vi "addSuccess.vi"(7 "execution time (sec)":dbl, 8 "error in (no error)":errorcluster, 10 "test":refnum<class>, 11 "TestResult in":refnum<class "TestResult.lvclass">) -> (0 "error out":errorcluster, 3 "TestResult in":refnum<class "TestResult.lvclass">)   [LabVIEW 2019, in "TestResult.lvclass"]
uses:
  TestResult.lvclass
  resultStatusChanged--Cluster.ctl
  resultStatus--enum.ctl
  TestResult.lvclass/TestResult.ctl
panel:
  # "JKI VI Tester for LabVIEW\nhttp://jkisoft.com/vi-tester\nCopyright (C) 2007-2009, JKI <info@jkisoft.com>\nALL RIGHTS RESERVED"
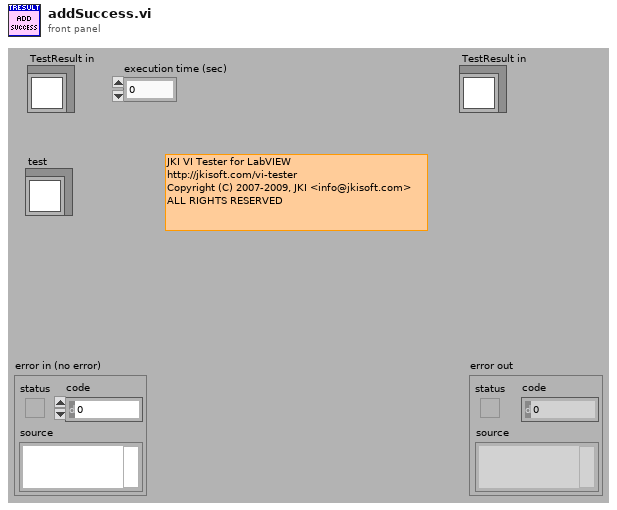
[diagram p1: front panel]
types:
  T1 = typedef "TestResult.lvclass/resultStatusChanged--Cluster.ctl" = cluster{"test":refnum<class>, "resultStatus":T2, "TestResult":refnum<class>, "test error":errorcluster, "execution time (sec)":dbl}
  T2 = typedef "TestResult.lvclass/resultStatus--enum.ctl" = enum16{"testPass", "testFailure", "testError", "testSkipped"}
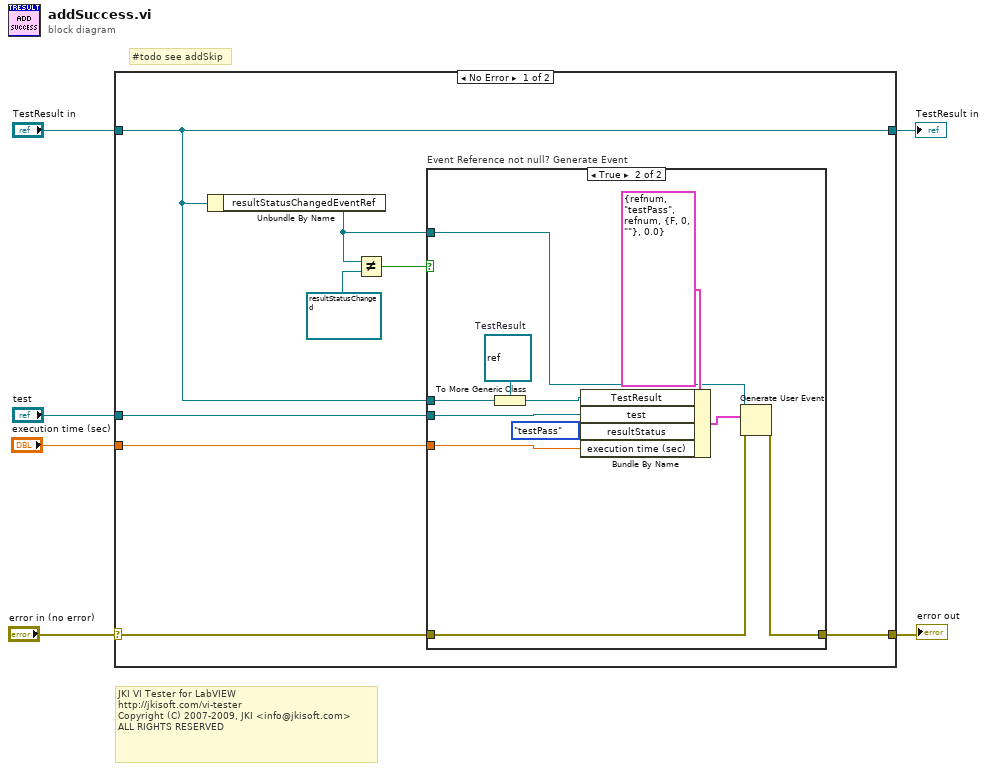
[diagram p0: block diagram]
diagram:
  # "#todo see addSkip"
  # "JKI VI Tester for LabVIEW\nhttp://jkisoft.com/vi-tester\nCopyright (C) 2007-2009, JKI <info@jkisoft.com>\nALL RIGHTS RESERVED"
  n1 = case shown="No Error" "error in (no error)" {
    selector: "error in (no error)" -> [w10 w28]
    tunnel: [w9 w28] -> w5
    tunnel: [w13 w27] -> w3
    tunnel: "TestResult in" -> [w13 w27]
    tunnel: "test" -> [w14 _]
    tunnel: "execution time (sec)" -> [w7 _]
    frame No Error {
      n2 = Unbundle By Name(w13) -> ("resultStatusChangedEventRef"=w12:refnum<user-event>)
      n3 = Not Equal?(x=w12, y=refnum<user-event> refnum ("resultStatusChangedEventRef")) -> (x != y?=w8:bool)
      n4 = case "Event Reference not null? Generate Event" shown="True" w8 {
        tunnel: w14 -> [_ w24]
        tunnel: w13 -> [_ w23]
        tunnel: w12 -> [_ w21]
        tunnel: w10 -> [w15 w20]
        tunnel: [w15 w19] -> w9
        tunnel: w7 -> [_ w16]
        frame False {
        }
        frame True {
          w17 = refnum<class> refnum  # TestResult
          n5 = To More Generic Class(target class=w17, reference=w23) -> (generic class reference=w18:refnum<class>)
          n6 = Bundle By Name(cluster=T1 {"test"=refnum, "resultStatus"=enum."testPass", "TestResult"=refnum, "test error"={"status"=FALSE, "code"=0, "source"=""}, "execution time (sec)"=0.0} ("event data"), "TestResult"=w18, "test"=w24, "resultStatus"=resultStatus--enum."testPass", "execution time (sec)"=w16) -> (w26:T1)
          n7 = Generate User Event(user event=w21, event data cluster=w26, error in=w20) -> (error out=w19:errorcluster)  [unwired: 1 in, 1 out]
        }
      }
    }
    frame Error {
    }
  }
  "error out" <- w5
  "TestResult in" <- w3
